vi "Centrized Error Handling.vi"(8 "error in (no error)":errorcluster, 9 "Error":errorcluster, 10 "Error Level":T1, 11 "Car Wash Controller in":refnum<class "Car Wash Controller.lvclass">) -> (0 "error out":errorcluster, 3 "Car Wash Controller out":refnum<class "Car Wash Controller.lvclass">)   [LabVIEW 2019, in "Car Wash Controller.lvlib" / "Car Wash Controller.lvclass"]
uses:
  Car Wash Controller.lvclass
  Error Level.ctl
  States -Enum.ctl
  Wash Steps.ctl
  Error Data.ctl
  Car Wash Controller Messages/Set State Msg/Set State Msg.lvclass
  <vilib>/ActorFramework/Actor/Actor.lvclass
  C:/Program Files (x86)/National Instruments/LabVIEW 2019/vi.lib/ActorFramework/Actor/Actor.lvclass
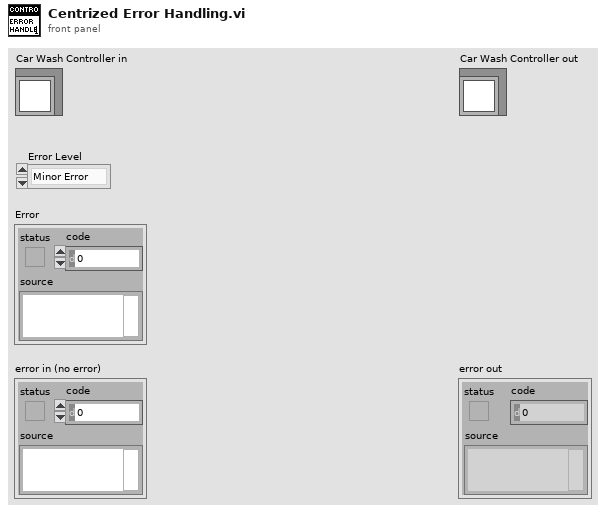
[diagram p1: front panel]
types:
  T1 = typedef "Car Wash Controller.lvlib/Car Wash Controller.lvclass/Error Level.ctl" = enum16{"Minor Error", "Wash Cycle Error", "System Error"}
  T2 = typedef "Car Wash Controller.lvlib/Car Wash Controller.lvclass/Error Data.ctl" = cluster{"Description":string, "Error Level":T1, "Time Stamp":timestamp, "State":T3, "Wash Steps":T4}
  T3 = typedef "Car Wash Controller.lvlib/Car Wash Controller.lvclass/States -Enum.ctl" = enum16{"Inital", "Wait for Start", "Start", "Wait for Vehicle Position", "Wash Step Execution", "Wash Step/Cycle Completion", "Wash Exit", "Wash Abort/Terminate State"}
  T4 = typedef "Car Wash Controller.lvlib/Car Wash Controller.lvclass/Wash Steps.ctl" = cluster{"Under Body Wash":bool, "Bug Remover":bool, "Pre-Soak":bool, "High Pressure Wash (Default)":bool, "Low Pressure Wax":bool, "Spot Free Rinse":bool, "Tire Shine Foam":bool, "Air Dry":bool}
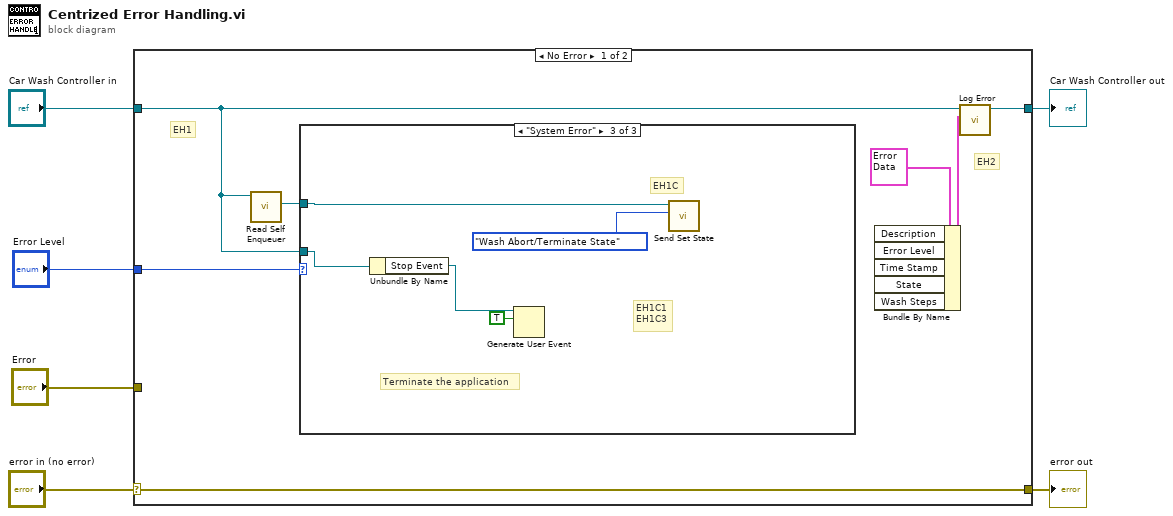
[diagram p0: block diagram]
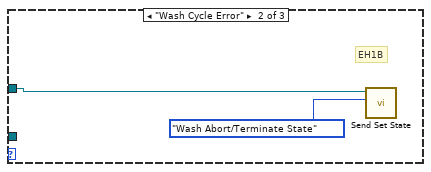
[diagram p3: hidden frame]
diagram:
  n1 = case shown="No Error" "error in (no error)" {
    selector: "error in (no error)" -> [w13 w22]
    tunnel: [w13 w22] -> w5
    tunnel: [w11 w21] -> w3
    tunnel: "Car Wash Controller in" -> [w7 w21]
    tunnel: "Error Level" -> [w12 _]
    tunnel: "Error" -> [_ _]
    frame No Error {
      # "EH2"
      # "EH1"
      n2 = call <vilib>:"Read Self Enqueuer.vi"("Actor"=w7) -> ("Self Enqueuer"=w8:refnum<class "Message Enqueuer.lvclass">)  [unwired: 10 in]
      n3 = case shown="\"System Error\"" w12 {
        tunnel: w8 -> [_ w15 w19]
        tunnel: w7 -> [_ _ w18]
        frame "Minor Error", Default {
          # "EH1A"
        }
        frame "Wash Cycle Error" {
          # "EH1B"
          n4 = call "Send Set State.vi"("State"=States_-Enum."Wash Abort/Terminate State", "Message Enqueuer"=w15) -> ()  [unwired: 8 in, 2 out]
        }
        frame "System Error" {
          # "EH1C1\nEH1C3"
          # "Terminate the application"
          # "EH1C"
          n5 = Unbundle By Name(w18) -> ("Stop Event"=w17:refnum<user-event>)
          n6 = Generate User Event(user event=w17, event data cluster=TRUE ("event data")) -> ()  [unwired: 2 in, 2 out]
          n7 = call "Send Set State.vi"("State"=States_-Enum."Wash Abort/Terminate State", "Message Enqueuer"=w19) -> ()  [unwired: 8 in, 2 out]
        }
      }
      n8 = Bundle By Name(cluster=T2 {"Description"="", "Error Level"=enum."Minor Error", "Time Stamp"=timestamp(0 s since 1904-01-01), "State"=enum."Inital", "Wash Steps"={"Under Body Wash"=FALSE, "Bug Remover"=FALSE, "Pre-Soak"=FALSE, "High Pressure Wash (Default)"=FALSE, "Low Pressure Wax"=FALSE, "Spot Free Rinse"=FALSE, "Tire Shine Foam"=FALSE, "Air Dry"=FALSE}} ("Error Data")) -> (w9:T2)  [unwired: 5 in]
      n9 = call "Log Error.vi"("Error Data"=w9, "Car Wash Controller in"=w7) -> ("Car Wash Controller out"=w11:refnum<class "Car Wash Controller.lvclass">)  [unwired: 8 in, 1 out]
    }
    frame Error {
    }
  }
  "error out" <- w5
  "Car Wash Controller out" <- w3
